vi "Offset Async Buffers.vi"(8 "error in (no error)":errorcluster, 10 "base Inline Buffer":refnum<class "Buffer.lvclass">, 11 "Framework in":refnum<class "Framework.lvclass">) -> (0 "error out":errorcluster, 3 "Framework out":refnum<class "Framework.lvclass">)   [LabVIEW 2019, in "DSF Core.lvlib" / "Framework.lvclass"]
uses:
  Framework.lvclass
  Buffer/Buffer.lvclass
  C:/Program Files (x86)/National Instruments/LabVIEW 2019/vi.lib/NI/Memory Manager/Classes/Pointer/Pointer.lvclass
  Framework.lvclass/Framework.ctl
  Interface/Dispatcher/Inline Buffer Parameters.ctl
  Interface/Plugin/Command Data.ctl
  Interface/Plugin/Command.ctl
  Interface/Plugin/Command Parameters.ctl
  <vilib>/NI/Memory Manager/Classes/Pointer/Pointer.lvclass/Pointer.ctl
  Interface/Plugin/Send Plugin Command.vi
  <vilib>/NI/Memory Manager/Classes/Pointer/Pointer.lvclass
  Interface/Dispatcher/Dispatcher Interface.lvclass
  Interface/Plugin/Plugin Interface.lvclass
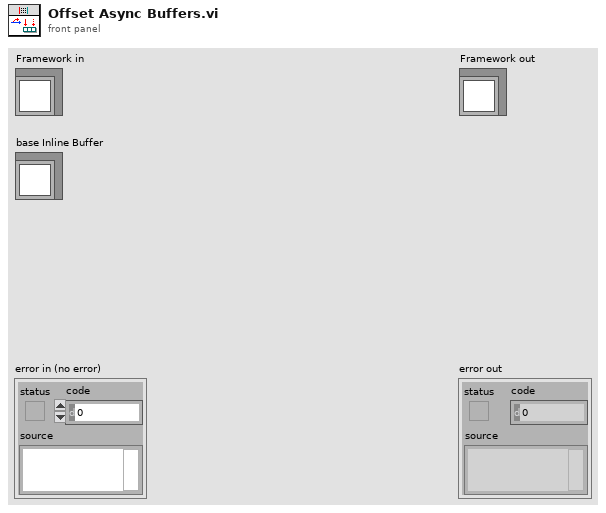
[diagram p1: front panel]
types:
  T1 = typedef "DSF Core.lvlib/Plugin Interface.lvclass/Command.ctl" = enum8{"Idle", "Start", "Set Inline Buffer", "Rx", "Tx", "Shutdown", "Error"}
  T2 = typedef "DSF Core.lvlib/Plugin Interface.lvclass/Command Parameters.ctl" = cluster{"arg1":u64, "arg2":u64}
  T3 = typedef "DSF Core.lvlib/Plugin Interface.lvclass/Command Data.ctl" = cluster{"Command":T1, "Parameters":T2}
  T4 = typedef "DSF Core.lvlib/Dispatcher Interface.lvclass/Inline Buffer Parameters.ctl" = cluster{"address":u64, "size":u64}
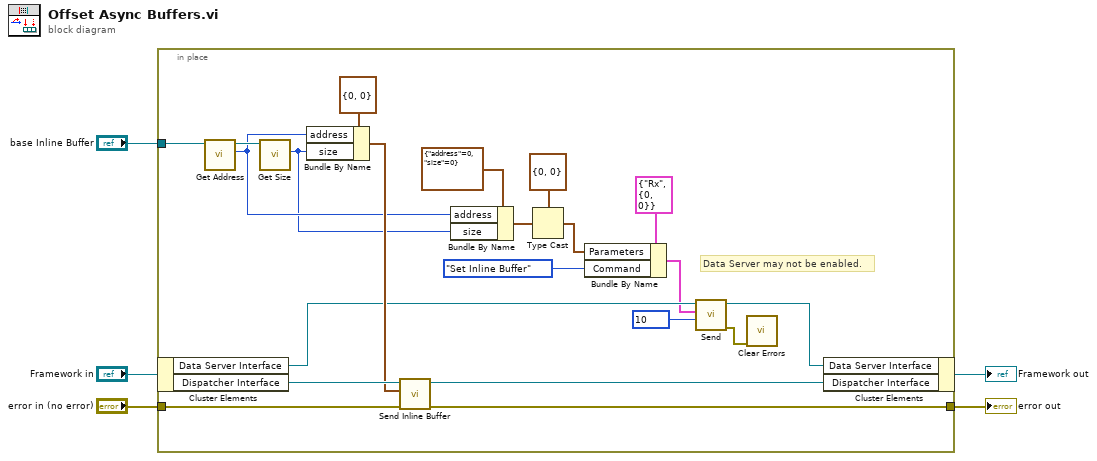
[diagram p0: block diagram]
diagram:
  n1 = in-place {
    in-place-border: "base Inline Buffer" -> [w26]
    in-place-border: "error in (no error)" -> [w23]
    in-place-border: [w6] -> w4
    # "Data Server may not be enabled."
    n2 = in-place-cluster #1("Framework in") -> ("Data Server Interface"=w12:refnum<class "Plugin Interface.lvclass">, "Dispatcher Interface"=w24:refnum<class "Dispatcher Interface.lvclass">)
    n3 = call <vilib>:"Get Address.vi"("Pointer in"=w26) -> ("address"=w10:u64, "Pointer out"=w25:refnum<class "Buffer.lvclass">)  [unwired: 9 in]
    n4 = call <vilib>:"Get Size.vi"("Pointer in"=w25) -> ("size"=w9:u64)  [unwired: 9 in, 1 out]
    n5 = Bundle By Name(cluster=T4 {"address"=0, "size"=0} ("Inline Buffer Parameters"), "address"=w10, "size"=w9) -> (w20:T4)
    n6 = call "Send Inline Buffer.vi"("error in (no error)"=w23, "Inline Buffer Parameters"=w20, "Dispatcher Interface in"=w24) -> ("error out"=w6:errorcluster, "Dispatcher Interface out"=w21:refnum<class "Dispatcher Interface.lvclass">)  [unwired: 7 in]
    n7 = Bundle By Name(cluster=cluster{"address":u64, "size":u64} {"address"=0, "size"=0}, "address"=w10, "size"=w9) -> (w17:cluster{"address":u64, "size":u64})
    n8 = Type Cast(type=T2 {"arg1"=0, "arg2"=0} ("Command Parameters"), x=w17) -> (*(type *) &x=w14:T2)
    n9 = Bundle By Name(cluster=T3 {"Command"=enum."Rx", "Parameters"={"arg1"=0, "arg2"=0}} ("command"), "Parameters"=w14, "Command"=Command."Set Inline Buffer") -> (w8:T3)
    n10 = call-poly "Send.vi"("timeout in ms (0)"=10, "command"=w8, "Plugin Interface in"=w12) -> ("error out"=w7:errorcluster, "Plugin Interface out"=w11:refnum<class "Plugin Interface.lvclass">)  [unwired: 7 in]
    n11 = call <vilib>:"Clear Errors.vi"("error in (no error)"=w7) -> ()  [unwired: 5 in, 2 out]
    n12 = in-place-cluster #1("Data Server Interface"=w11, "Dispatcher Interface"=w21) -> (→"Framework out":refnum<class "Framework.lvclass">)
  }
  "error out" <- w4
